vi "Post-Build Action.vi"(5 "Files Generated by Build":path[](array[path]), 6 "Top Level/Always Included VIs":path[](array[path]), 7 "Destination Path":path, 8 "error in (no error)":errorcluster, 9 "Target Name":string, 10 "Build Specification Name":string, 11 "Project Path":path) -> (0 "error out":errorcluster)   [LabVIEW 2014]
panel:
  in  "illegalCharacers":string[](array[string])=[".lvproj", " ", "/", "\\", ":", "*", "?", "\"", "<", ">", "|"]
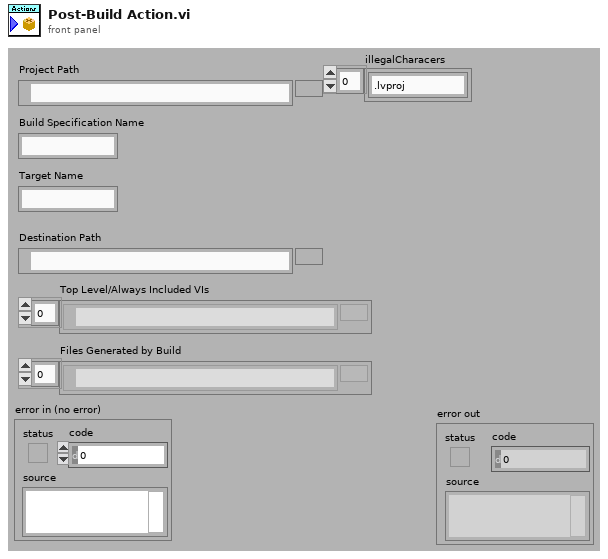
[diagram p1: front panel]
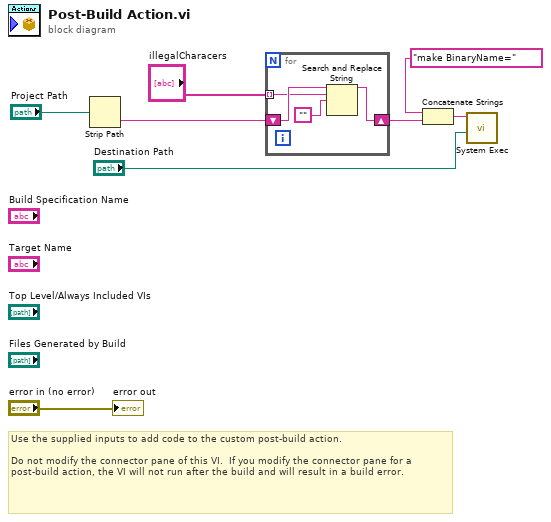
[diagram p0: block diagram]
diagram:
  # "Use the supplied inputs to add code to the custom post-build action.\n\nDo not modify the connector pane of this VI.  If you modify the connector pane for a post-build action, the VI will not run after the build and will result in a build error."
  n1 = Strip Path(path="Project Path") -> (name=w4:string)  [unwired: 1 out]
  n2 = for {
    tunnel: "illegalCharacers" -> [w10] mode=indexing
    shift-right: [w9] -> w1
    shift-left: w4 -> [w11]
    n3 = Search and Replace String(input string=w11, search string=w10, replace string="") -> (result string=w9:string)  [unwired: 5 in, 3 out]
  }
  n4 = Concatenate Strings("make BinaryName=" ("command line"), w1) -> (w2:string)
  n5 = call <vilib>:"System Exec.vi"("working directory"="Destination Path", "command line"=w2) -> ()  [unwired: 6 in, 4 out]
  "error out" <- "error in (no error)"
